vi "Trapezoidal Velocity Profile.vi"(8 "t":dbl format="%#_13g", 9 "axis displacement (distance)":dbl format="%#_13g", 10 "initial velocity":dbl format="%#_13g", 11 "set velocity":dbl format="%#_13g") -> (2 "velocity profile at t":dbl)   [LabVIEW 2016]
panel:
  in  "max acceleration":dbl format="%#_13g"
  in  "max velocity":dbl format="%#_13g"
  # "input"
  # "parameters"
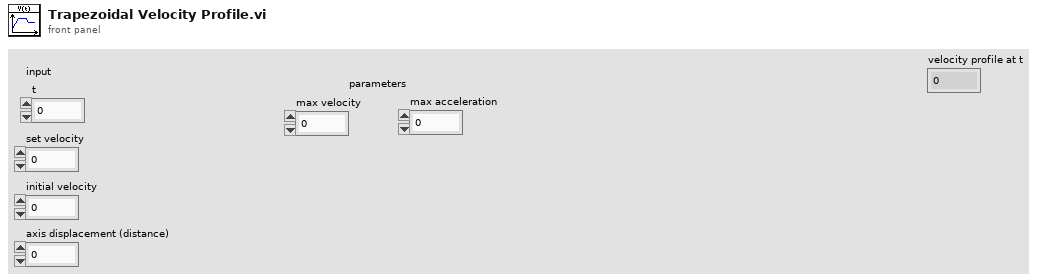
[diagram p1: front panel]
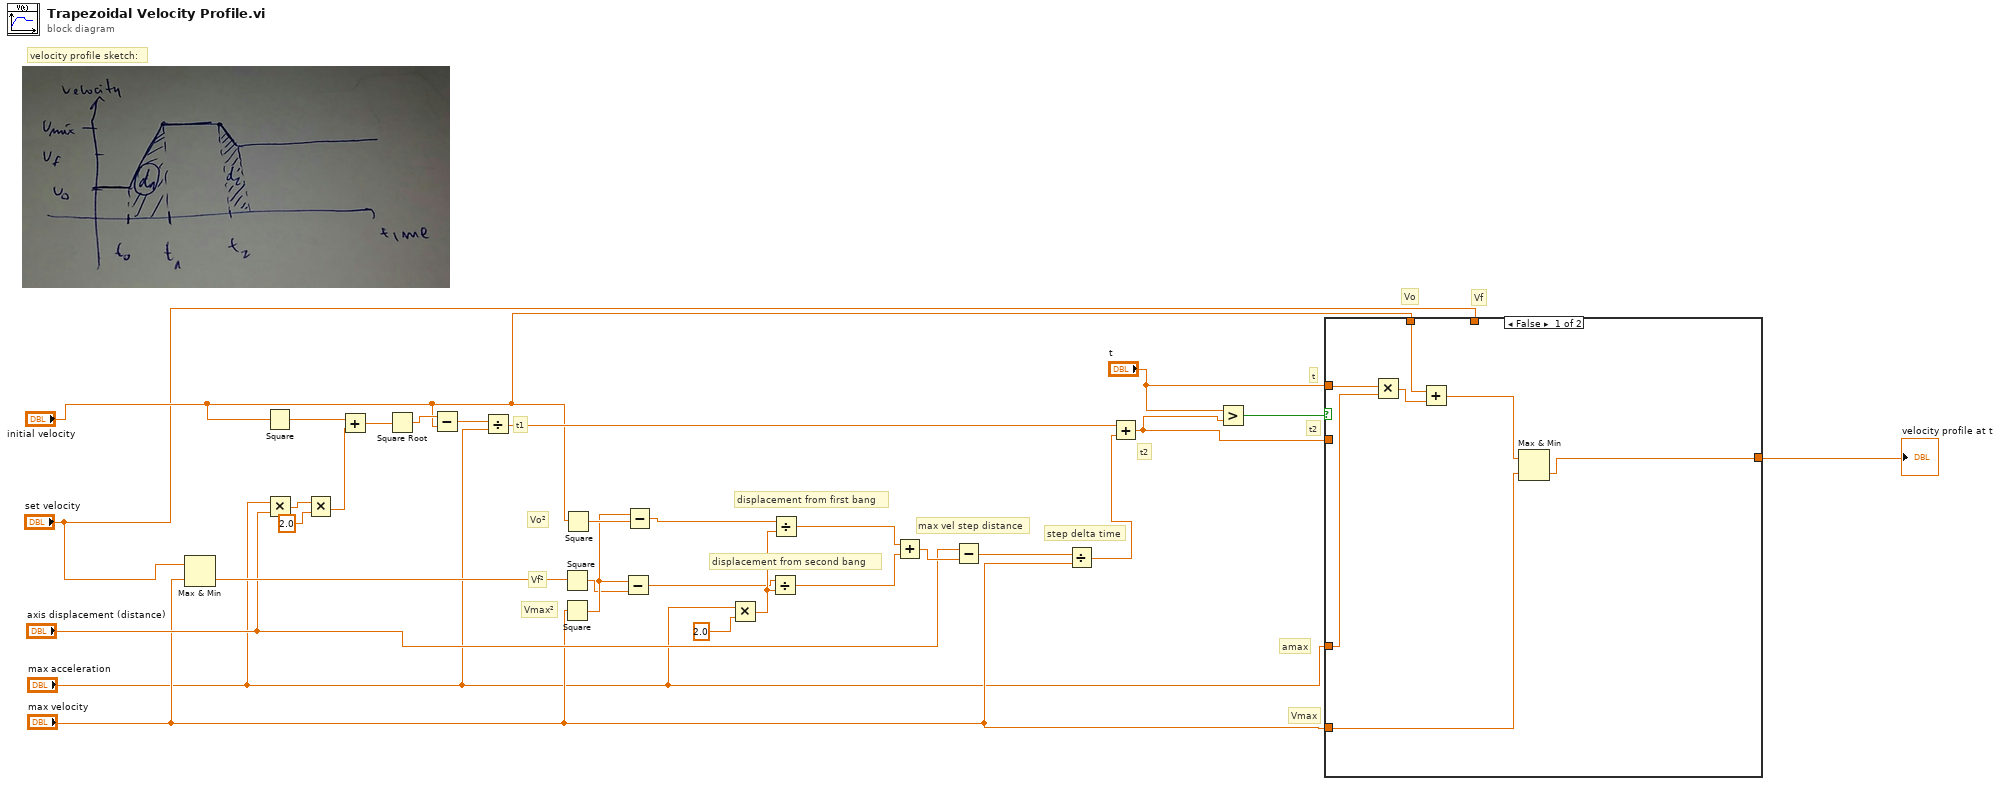
[diagram p0: block diagram]
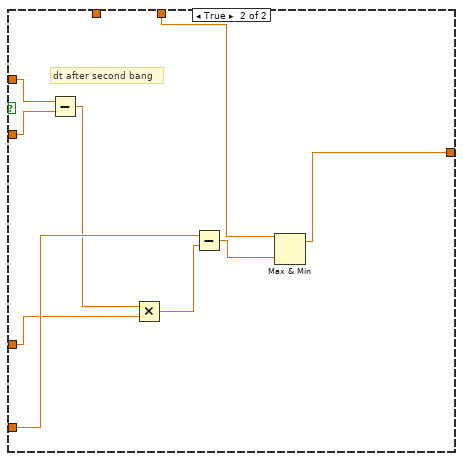
[diagram p2: hidden frame]
diagram:
  # "amax"
  # "Vmax"
  # "t2"
  # "t"
  # "Vo"
  # "Vf"
  # "t2"
  # "step delta time"
  # "max vel step distance"
  # "velocity profile sketch:"
  # "displacement from second bang"
  # "displacement from first bang"
  # "Vo²"
  # "Vf²"
  # "Vmax²"
  # "t1"
  n1 = Max & Min(x="set velocity", y="max velocity") -> (min(x,y)=w16:dbl)  [unwired: 1 out]
  n2 = Square(x="initial velocity") -> (x^2=w28:dbl)
  n3 = Multiply(x="max acceleration", y="axis displacement (distance)") -> (x*y=w30:dbl)
  n4 = Multiply(x=w30, y=2.0) -> (x*y=w27:dbl)
  n5 = Add(x=w28, y=w27) -> (x+y=w26:dbl)
  n6 = Square Root(x=w26) -> (sqrt(x)=w25:dbl)
  n7 = Subtract(x=w25, y="initial velocity") -> (x-y=w24:dbl)
  n8 = Divide(x=w24, y="max acceleration") -> (x/y=w11:dbl)
  n9 = Square(x=w16) -> (x^2=w21:dbl)
  n10 = Square(x="max velocity") -> (x^2=w22:dbl)
  n11 = Square(x="initial velocity") -> (x^2=w23:dbl)
  n12 = Subtract(x=w22, y=w21) -> (x-y=w17:dbl)
  n13 = Subtract(x=w22, y=w23) -> (x-y=w19:dbl)
  n14 = Multiply(x="max acceleration", y=2.0) -> (x*y=w18:dbl)
  n15 = Divide(x=w17, y=w18) -> (x/y=w14:dbl)
  n16 = Divide(x=w19, y=w18) -> (x/y=w15:dbl)
  n17 = Add(x=w15, y=w14) -> (x+y=w13:dbl)
  n18 = Subtract(x="axis displacement (distance)", y=w13) -> (x-y=w12:dbl)
  n19 = Divide(x=w12, y="max velocity") -> (x/y=w10:dbl)
  n20 = Add(x=w11, y=w10) -> (x+y=w3:dbl)
  n21 = Greater?(x="t", y=w3) -> (0:w9:bool)
  n22 = case shown="False" w9 {
    tunnel: "t" -> [w37 w44]
    tunnel: "initial velocity" -> [w35 _]
    tunnel: "max acceleration" -> [w36 w45]
    tunnel: "max velocity" -> [w32 w46]
    tunnel: [w31 w38] -> w1
    tunnel: "set velocity" -> [_ w40]
    tunnel: w3 -> [_ w43]
    frame False {
      n23 = Multiply(x=w37, y=w36) -> (x*y=w34:dbl)
      n24 = Add(x=w35, y=w34) -> (x+y=w33:dbl)
      n25 = Max & Min(x=w33, y=w32) -> (min(x,y)=w31:dbl)  [unwired: 1 out]
    }
    frame True {
      # "dt after second bang"
      n26 = Subtract(x=w44, y=w43) -> (x-y=w42:dbl)
      n27 = Multiply(x=w42, y=w45) -> (x*y=w41:dbl)
      n28 = Subtract(x=w46, y=w41) -> (x-y=w39:dbl)
      n29 = Max & Min(x=w40, y=w39) -> (max(x,y)=w38:dbl)  [unwired: 1 out]
    }
  }
  "velocity profile at t" <- w1
